vi "RunWavesCont.vi"(6 "Analogue Out":waveform(dbl)[](array[waveform]), 7 "Digital Out":digitalwaveform[](array[waveform]), 9 "Microscope Settings":T1={"Mode"=enum."X", "Slit"={"Scanning Mode"=0.0, "Slit Width /%"=0.0}, "Colour"=[], "Focus Offset /um"=0.0, "Exposure/ms"=0.0, "Piezo Position /um"=0.0, "ROI"={"X"={"Start /px"=0.0, "Step /px"=0.0, "Range /px"=0.0}, "Y"={"Start /px"=0.0, "Step /px"=0.0, "Range /px"=0.0}, "Z "={"Start /um"=0.0, "Step/um"=0.0, "Range /um"=0.0}, "T "={"Start /s"=0.0, "Step /s"=0.0, "Range /s"=0.0}}, "Samples per millisecond"=0.0, "Relax/ms"=0.0, "Readout Direction"=0.0, "Trigger Source"=0.0, "Camera Delay /ms"=0.0, "Under Scan /ms"=0.0, "Slit Delay"=100.0, "Waveforms"={"Analogue Out"=[], "Digital Out"=[]}} {"Focus Offset /um" scale=-2.0..2.0 scale format="%.2f"; "Under Scan /ms" min=0.0 max=10.0 step=0.05; "ROI"."T"."Range /s" min=0.0 max=10.0 step=0.05; "ROI"."T"."Step /s" min=0.0 max=10.0 step=0.05; "ROI"."T"."Start /s" min=0.0 max=10.0 step=0.05; "ROI"."X"."Range /px" min=0.0 max=10.0 step=0.05; "ROI"."X"."Step /px" min=0.0 max=10.0 step=0.05; "ROI"."X"."Start /px" min=0.0 max=10.0 step=0.05; "ROI"."Y"."Range /px" min=0.0 max=10.0 step=0.05; "ROI"."Y"."Step /px" min=0.0 max=10.0 step=0.05; "ROI"."Y"."Start /px" min=0.0 max=10.0 step=0.05; "ROI"."Z"."Range /um" min=0.0 max=10.0 step=0.05; "ROI"."Z"."Step/um" min=0.0 max=10.0 step=0.05; "ROI"."Z"."Start /um" min=0.0 max=10.0 step=0.05; "Colour"."Colour"."Filter" items=["Empty"=1, ""=2, ""=3, "561"=4, ""=5, "488"=6]; "Camera Delay /ms" min=0.0 max=10.0 step=0.05; "Trigger Source" items=["Internal"=1.0, "External"=2.0]; "Readout Direction" items=["Internal"=1.0, "External"=2.0]; "Slit"."Scanning Mode" items=["Full Frame"=1.0, "Slit Scanning"=12.0]; "Piezo Position /um" min=0.0 max=10.0 step=0.05; "Exposure/ms" min=0.0 max=10.0 step=0.05; "Relax/ms" min=1.0 max=2.0 step=1.0}, 10 "Digital In":refnum<k21>, 11 "Analogue  in":refnum<k21>) -> (2 "Digital Out":refnum<k21>, 3 "Analogue Out":refnum<k21>)   [LabVIEW 2016]
uses:
  controls/Microscope Settings.ctl
  controls/ColourCalibration.ctl
  <vilib>/DAQmx/write.llb/DAQmx Write (Digital 1D Wfm NChan NSamp).vi
  <vilib>/DAQmx/write.llb/DAQmx Write (Analog 1D Wfm NChan NSamp).vi
  <vilib>/Waveform/WDTOps.llb/WDT Number of Waveform Samples DBL.vi
  <vilib>/DAQmx/configure/timing.llb/DAQmx Timing (Sample Clock).vi
  <vilib>/Waveform/DWDTOps.llb/DWDT Uncompress Digital.vi
  <vilib>/DAQmx/miscellaneous.llb/DAQmx Fill In Error Info.vi
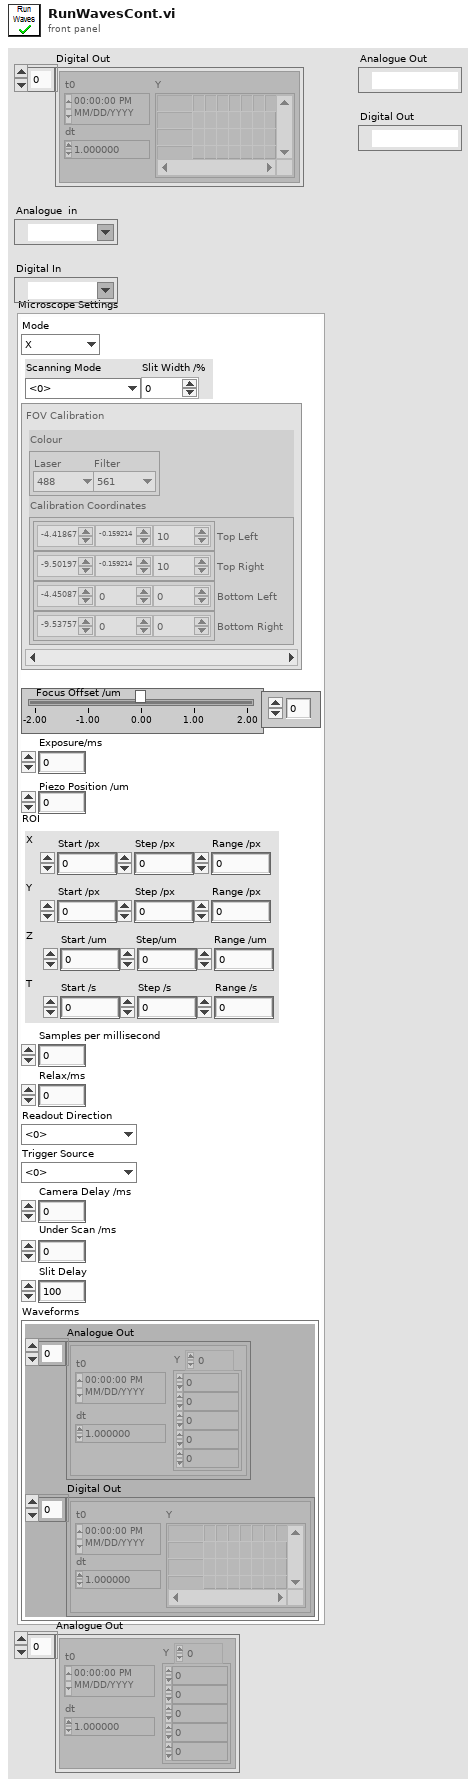
[diagram p1: front panel]
types:
  T1 = typedef "Microscope Settings.ctl" = cluster{"Mode":enum16{"Brightfield", "X", "XY", "XYZ", "XYZT", "XYZC", "Tweezers", "Virus"}, "Slit":cluster{"Scanning Mode":dbl, "Slit Width /%":dbl}, "Colour":T2, "Focus Offset /um":dbl, "Exposure/ms":dbl, "Piezo Position /um":dbl, "ROI":cluster{"X":cluster{"Start /px":dbl, "Step /px":dbl, "Range /px":dbl}, "Y":cluster{"Start /px":dbl, "Step /px":dbl, "Range /px":dbl}, "Z ":cluster{"Start /um":dbl, "Step/um":dbl, "Range /um":dbl}, "T ":cluster{"Start /s":dbl, "Step /s":dbl, "Range /s":dbl}}, "Samples per millisecond":dbl, "Relax/ms":dbl, "Readout Direction":dbl, "Trigger Source":dbl, "Camera Delay /ms":dbl, "Under Scan /ms":dbl, "Slit Delay":dbl, "Waveforms":cluster{"Analogue Out":waveform(dbl)[], "Digital Out":digitalwaveform[]}}
  T2 = typedef "ColourCalibration.ctl" = cluster{"Colour":cluster{"Laser":enum16{"Brightfield", "445", "488", "561", "647"}, "Filter":u16}, "Calibration Coordinates":cluster{"Top Left":dbl[], "Top Right":dbl[], "Bottom Left":dbl[], "Bottom Right":dbl[]}}[]
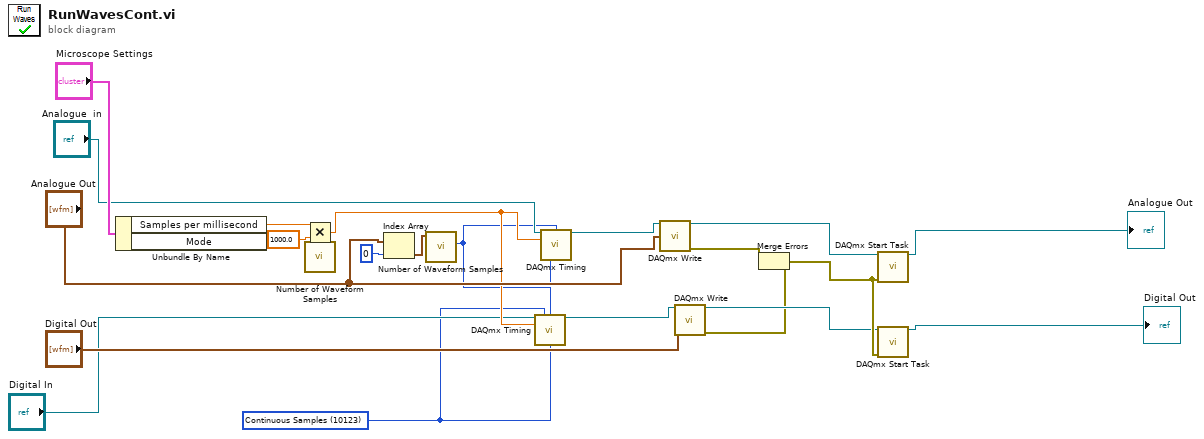
[diagram p0: block diagram]
diagram:
  w1 = 10123 items=["Finite Samples"=10178, "Continuous Samples"=10123, "Hardware Timed Single Point"=12522] ("sample mode")
  n1 = Unbundle By Name("Microscope Settings") -> ("Samples per millisecond"=w5:dbl)  [unwired: 1 out]
  n2 = Multiply(x=w5, y=1000.0) -> (x*y=w11:dbl)
  n3 = call-poly <vilib>:"Number of Waveform Samples.vi"() -> ()  [unwired: 9 in, 3 out]
  n4 = Index Array(array="Analogue Out", index=0) -> (element=w7:waveform(dbl))
  n5 = call-poly <vilib>:"Number of Waveform Samples.vi"("waveform in"=w7) -> ("number of samples"=w8:i32)  [unwired: 8 in, 2 out]
  n6 = call-poly <vilib>:"DAQmx Timing.vi"("task/channels in"="Digital In", "sample mode"=w1, "samples per channel"=w8, "rate"=w11) -> ("task out"=w13:refnum<k21>)  [unwired: 10 in, 1 out]
  n7 = call-poly <vilib>:"DAQmx Timing.vi"("task/channels in"="Analogue  in", "sample mode"=w1, "samples per channel"=w8, "rate"=w11) -> ("task out"=w12:refnum<k21>)  [unwired: 10 in, 1 out]
  n8 = call-poly <vilib>:"DAQmx Write.vi"("task/channels in"=w12, "data"="Analogue Out") -> ("task out"=w16:refnum<k21>, "error out"=w14:errorcluster)  [unwired: 11 in, 1 out]
  n9 = call-poly <vilib>:"DAQmx Write.vi"("task/channels in"=w13, "data"="Digital Out") -> ("task out"=w17:refnum<k21>, "error out"=w15:errorcluster)  [unwired: 11 in, 1 out]
  n10 = Merge Errors(w14, w15) -> (w18:errorcluster)
  n11 = call <vilib>:"DAQmx Start Task.vi"("task/channels in"=w16, "error in"=w18) -> ("task out"=→"Analogue Out":refnum<k21>)  [unwired: 12 in, 1 out]
  n12 = call <vilib>:"DAQmx Start Task.vi"("task/channels in"=w17, "error in"=w18) -> ("task out"=→"Digital Out":refnum<k21>)  [unwired: 12 in, 1 out]
